vi "Shoot preset find corresponding RPM.vi"(1 "Shooter Preset speeds (RPM)":T1=enum."Target Zone") -> (0 "Shooter Speed (RPM)":dbl)   [LabVIEW 2019]
uses:
  Shooter Preset speeds Type Def.ctl
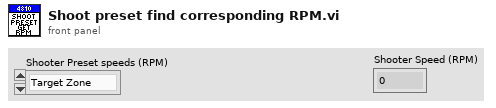
[diagram p1: front panel]
types:
  T1 = typedef "Shooter Preset speeds Type Def.ctl" = enum16{"Not Applicable", "Target Zone", "Initiation Line", "Close end of Trench Run", "Control Panel"}
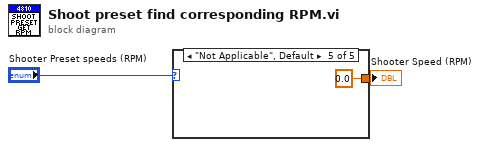
[diagram p0: block diagram]
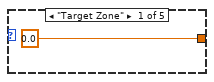
[diagram p2: hidden frame]
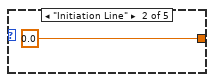
[diagram p3: hidden frame]
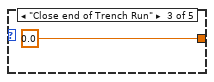
[diagram p4: hidden frame]
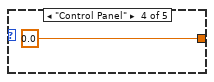
[diagram p5: hidden frame]
diagram:
  n1 = case shown="\"Not Applicable\", Default" "Shooter Preset speeds (RPM)" {
    tunnel: [0.0 ("Shooter Speed (RPM)") 0.0 ("Shooter Speed (RPM)") 0.0 ("Shooter Speed (RPM)") 0.0 ("Shooter Speed (RPM)") 0.0 ("Shooter Speed (RPM)")] -> w1
    frame "Target Zone" {
    }
    frame "Initiation Line" {
    }
    frame "Close end of Trench Run" {
    }
    frame "Control Panel" {
    }
    frame "Not Applicable", Default {
    }
  }
  "Shooter Speed (RPM)" <- w1
